vi "ExtractDeviceInfo.vi"(0 "Line IN":string) -> (1 "valid record?":bool, 2 "Device Info":T1={"Sensor Serial No.:"="", "Wafer:"="", "Batch:"="", "Manufacturer:"="Hamamatsu", "Device Category:"="ATLAS18SS", "Database Serial No.:"="", "Institution"="", "Current Location"="", "Assembled?"=FALSE, "Component:"="SENSOR"})   [LabVIEW 2013]
uses:
  <vilib>/regexp/Match Regular Expression.xnode
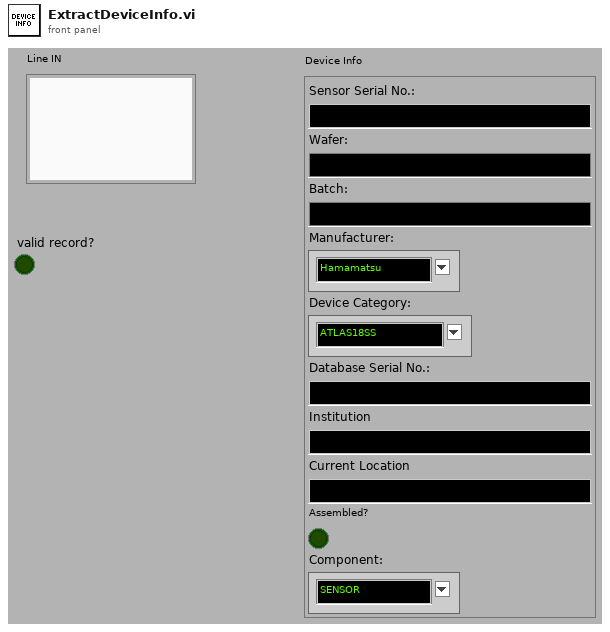
[diagram p1: front panel]
types:
  T1 = cluster{"Sensor Serial No.:":string, "Wafer:":string, "Batch:":string, "Manufacturer:":string, "Device Category:":string, "Database Serial No.:":string, "Institution":string, "Current Location":string, "Assembled?":bool, "Component:":string}
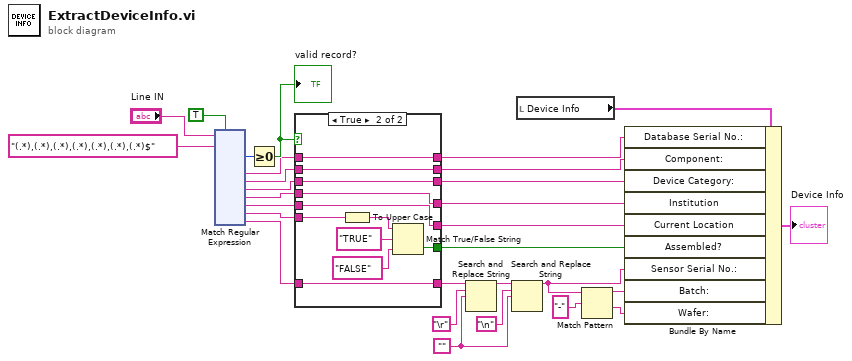
[diagram p0: block diagram]
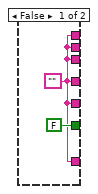
[diagram p2: hidden frame]
diagram:
  w4 = ""
  n1 = xnode "Match Regular Expression"("input string"="Line IN", "regular expression"="(.*),(.*),(.*),(.*),(.*),(.*),(.*)$", "ignore case? (F)"=TRUE) -> ("offset past match"=w26:i32, "submatch 1"=w24:string, "submatch 2"=w23:string, "submatch 3"=w22:string, "submatch 4"=w21:string, "submatch 5"=w20:string, "submatch 6"=w19:string, "submatch 7"=w7:string)  [unwired: 3 in, 4 out]
  n2 = Greater Or Equal To 0?(x=w26) -> (x >= 0?=w25:bool)
  "valid record?" <- w25
  n3 = case shown="True" w25 {
    tunnel: w24 -> [_ w42]
    tunnel: [w30 w42] -> w12
    tunnel: w23 -> [_ w41]
    tunnel: [w30 w41] -> w11
    tunnel: w22 -> [_ w40]
    tunnel: [w30 w40] -> w10
    tunnel: w21 -> [_ w39]
    tunnel: [w30 w39] -> w9
    tunnel: w20 -> [_ w38]
    tunnel: [w30 w38] -> w8
    tunnel: w19 -> [_ w37]
    tunnel: [FALSE ("selection") w33] -> w16
    tunnel: w7 -> [_ w32]
    tunnel: [w30 w32] -> w3
    frame False {
      w30 = ""
    }
    frame True {
      n4 = To Upper Case(1:w37) -> (0:w36:string)
      n5 = Match True/False String(2:"FALSE" ("false string"), 3:"TRUE" ("true string"), 4:w36) -> (0:w33:bool)  [unwired: 1 out]
    }
  }
  n6 = Search and Replace String(input string=w3, search string="\r", replace string=w4) -> (result string=w2:string)  [unwired: 5 in, 3 out]
  n7 = Search and Replace String(input string=w2, search string="\n", replace string=w4) -> (result string=w1:string)  [unwired: 5 in, 3 out]
  n8 = local read "Device Info"() -> (w17:T1)
  n9 = Match Pattern(string=w1, regular expression="-") -> (before substring=w14:string, after substring=w13:string)  [unwired: 1 in, 2 out]
  n10 = Bundle By Name(cluster=w17, "Database Serial No.:"=w12, "Component:"=w11, "Device Category:"=w10, "Institution"=w9, "Current Location"=w8, "Assembled?"=w16, "Sensor Serial No.:"=w1, "Batch:"=w14, "Wafer:"=w13) -> (→"Device Info":T1)
